vi "Avocent_send_cmd.vi"(8 "error in":errorcluster, 9 "timeout ms":i32=6000, 10 "Avocent IP (in)":string, 11 "HTTP command":string) -> (0 "error out":errorcluster, 2 "Avocent IP (out)":string, 3 "Replay":string)   [LabVIEW 2020]
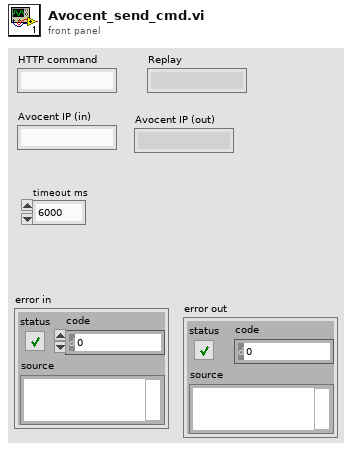
[diagram p1: front panel]
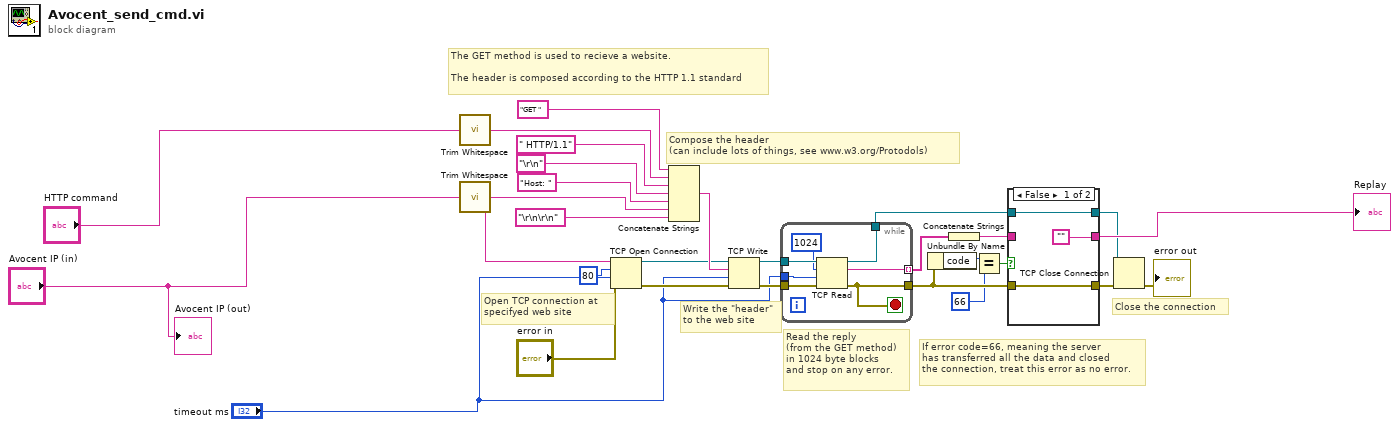
[diagram p0: block diagram]
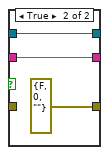
[diagram p2: hidden frame]
diagram:
  # "Compose the header\n(can include lots of things, see www.w3.org/Protodols)"
  # "The GET method is used to recieve a website.\n\nThe header is composed according to the HTTP 1.1 standard"
  # "Close the connection"
  # "If error code=66, meaning the server\nhas transferred all the data and closed\nthe connection, treat this error as no error."
  # "Read the reply\n(from the GET method)\nin 1024 byte blocks\nand stop on any error."
  # "Write the \"header\"\nto the web site"
  # "Open TCP connection at\nspecifyed web site"
  n1 = call <vilib>:"Trim Whitespace.vi"("string"="HTTP command") -> ("trimmed string"=w26:string)  [unwired: 1 in]
  n2 = call <vilib>:"Trim Whitespace.vi"("string"="Avocent IP (in)") -> ("trimmed string"=w27:string)  [unwired: 1 in]
  n3 = TCP Open Connection(address=w27, remote port or service name=u16 80 ("remote port"), timeout ms (60000)="timeout ms", error in (no error)="error in") -> (connection ID=w6:refnum<k5>, error out=w5:errorcluster)  [unwired: 1 in]
  n4 = Concatenate Strings("GET " ("Command"), w26, " HTTP/1.1" ("Command"), "\r\n" ("string"), "Host: " ("Command"), w27, "\r\n\r\n" ("string")) -> (w24:string)
  n5 = TCP Write(connection ID=w6, data in=w24, error in (no error)=w5, 9:"timeout ms") -> (connection ID out=w9:refnum<k5>, error out=w10:errorcluster)  [unwired: 1 out]
  n6 = while {
    tunnel: w10 -> [w35]
    tunnel: w9 -> [w34]
    tunnel: [w30] -> w12
    tunnel: [w33] -> w15
    tunnel: [w32] -> w13 mode=indexing
    tunnel: "timeout ms" -> [w29]
    stop <- w30 stop-if-true
    n7 = TCP Read(connection ID=w34, bytes to read=1024, error in (no error)=w35, 9:w29) -> (connection ID out=w33:refnum<k5>, data out=w32:string, error out=w30:errorcluster)  [unwired: 1 in]
  }
  n8 = Unbundle By Name(w12) -> ("code"=w7:i32)
  n9 = Concatenate Strings(w13) -> (w14:string)
  n10 = Equal?(x=w7, y=66) -> (x = y?=w8:bool)
  n11 = case shown="False" w8 {
    tunnel: ["" w40] -> w19
    tunnel: w14 -> [_ w40]
    tunnel: [w37 errorcluster {"status"=FALSE, "code"=0, "source"=""} ("error in (no error)")] -> w17
    tunnel: w12 -> [w37 _]
    tunnel: w15 -> [w36 w39]
    tunnel: [w36 w39] -> w16
    frame False {
    }
    frame True {
    }
  }
  "Replay" <- w19
  n12 = TCP Close Connection(connection ID=w16, error in (no error)=w17) -> (error out=→"error out":errorcluster)  [unwired: 1 in, 1 out]
  "Avocent IP (out)" <- "Avocent IP (in)"
